vi "DIO Averager.vi"(1 "In":bool, 2 "Number of Cycles to average":i32) -> (0 "Out":bool)   [LabVIEW 2014]
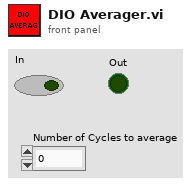
[diagram p1: front panel]
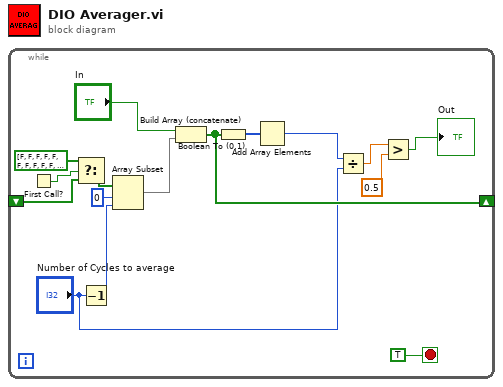
[diagram p0: block diagram]
diagram:
  n1 = while {
    shift-right: [w9] -> _
    shift-left: _ -> [w3]
    stop <- TRUE stop-if-true
    n2 = First Call?() -> (First Call?: T/F=w1:bool)
    n3 = Select(t=bool[] [FALSE, FALSE, FALSE, FALSE, FALSE, FALSE, FALSE, FALSE, FALSE, FALSE, FALSE, FALSE, FALSE, FALSE, FALSE, FALSE, FALSE, FALSE, FALSE, FALSE, FALSE, FALSE, FALSE, FALSE, FALSE, FALSE, FALSE, FALSE, FALSE, FALSE, FALSE, FALSE, FALSE, FALSE, FALSE, FALSE, FALSE, FALSE, FALSE, FALSE, FALSE, FALSE, FALSE, FALSE, FALSE, FALSE, FALSE, FALSE, FALSE, FALSE, FALSE, FALSE, FALSE, FALSE, FALSE, FALSE, FALSE, FALSE, FALSE, FALSE, FALSE, FALSE, FALSE, FALSE, FALSE, FALSE, FALSE, FALSE, FALSE, FALSE, FALSE, FALSE, FALSE, FALSE, FALSE, FALSE, FALSE, FALSE, FALSE, FALSE, FALSE, FALSE, FALSE, FALSE, FALSE, FALSE, FALSE, FALSE, FALSE, FALSE, FALSE, FALSE, FALSE, FALSE, FALSE, FALSE, FALSE, FALSE, FALSE, FALSE, TRUE], s=w1, f=w3) -> (s? t:f=w4:bool[])
    n4 = Decrement(x="Number of Cycles to average") -> (x-1=w6:i32)
    n5 = Array Subset(array=w4, index=0, length=w6) -> (w8:bool[])
    n6 = Build Array (concatenate)("In", w8) -> (w9:bool[])
    n7 = Boolean To (0,1)(Boolean=w9) -> (0, 1=w11:i16[])
    n8 = Add Array Elements(numeric array=w11) -> (sum=w10:i16)
    n9 = Divide(x=w10, y="Number of Cycles to average") -> (x/y=w15:dbl)
    n10 = Greater?(x=w15, y=0.5) -> (0:→"Out":bool)
  }
